vi "ERD_Event_Trigger.vi"(0 ".NET Refnum in":refnum<k24>, 5 "GEA Inputs":T1 {"Destination" format="%.0x"; "Source" format="%.0x"}, 9 "ERD Number":u16, 11 "error in (no error)":errorcluster) -> (4 ".NET Refnum out":refnum<k24>, 15 "error out":errorcluster)   [LabVIEW 2016]
uses:
  Common/LabVIEW GEA2 Toolkit/LabVIEW_GEA2_Toolkit.lvlibp/type defs/Source_Destination.ctl
  Q:/Common/DLLs/GEA3/GeaCommunication.dll
  Common/DLLs/GEA3/GeaCommunication.dll
  Common/LabVIEW GEA2 Toolkit/LabVIEW_GEA2_Toolkit.lvlibp/type defs/ERD Read Data In.ctl
  Common/LabVIEW GEA2 Toolkit/LabVIEW_GEA2_Toolkit.lvlibp/type defs/Data Type.ctl
  Common/LabVIEW GEA2 Toolkit/LabVIEW_GEA2_Toolkit.lvlibp/type defs/ERD Write Data In.ctl
  Common/LabVIEW GEA2 Toolkit/LabVIEW_GEA2_Toolkit.lvlibp
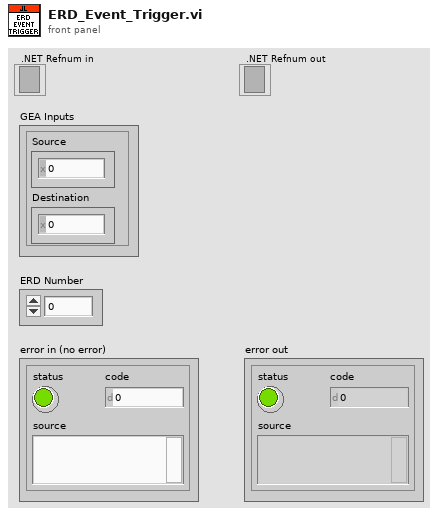
[diagram p1: front panel]
types:
  T1 = typedef "LabVIEW_GEA2_Toolkit.lvlibp/Source_Destination.ctl" = cluster{"Source":u8, "Destination":u8}
  T2 = typedef "LabVIEW_GEA2_Toolkit.lvlibp/ERD Write Data In.ctl" = cluster{"ERD Number":u16, "Data Type":T3, "Data":string}
  T3 = typedef "LabVIEW_GEA2_Toolkit.lvlibp/Data Type.ctl" = enum16{"string", "boolean", "uint8_t", "uint16_t", "uint32_t", "uint64_t", "int8_t", "int16_t", "int32_t", "int64_t"}
  T4 = typedef "LabVIEW_GEA2_Toolkit.lvlibp/ERD Read Data In.ctl" = cluster{"ERD Number":u16, "Data Type":T3}
  T5 = typedef "LabVIEW_GEA2_Toolkit.lvlibp/ERD Read Data Out.ctl" = cluster{"ERD Number":u16, "Data":string}
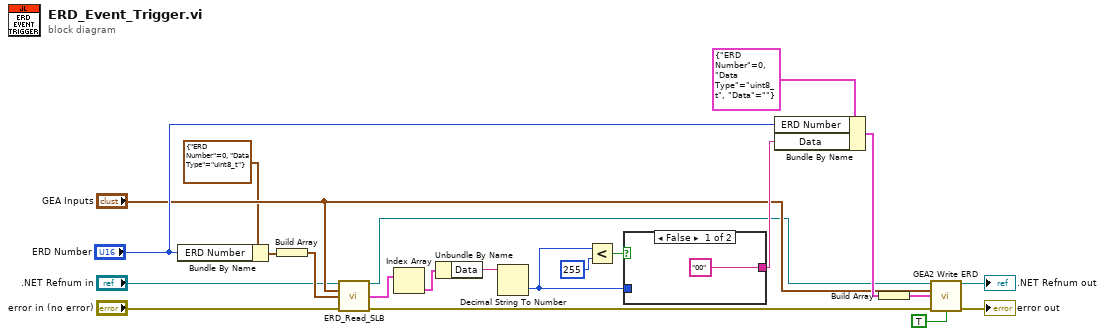
[diagram p0: block diagram]
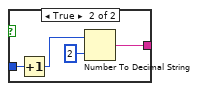
[diagram p2: hidden frame]
diagram:
  n1 = Bundle By Name(cluster=T4 {"ERD Number"=0, "Data Type"=enum."uint8_t"} ("ERD Read Data In"), "ERD Number"="ERD Number") -> (w8:T4)
  n2 = Build Array(w8) -> (w9:T4[])
  n3 = call "ERD_Read_SLB.vi"("GEA2 Reference In"=".NET Refnum in", "GEA Inputs"="GEA Inputs", "Read ERD List"=w9, "Error In"="error in (no error)") -> ("GEA2 Reference Out"=w16:refnum<k24>, "ERD Data Out"=w10:T5[], "Error Out"=w13:errorcluster)  [unwired: 9 in]
  n4 = Index Array(array=w10) -> (element=w11:T5)  [unwired: 1 in]
  n5 = Unbundle By Name(w11) -> ("Data"=w12:string)
  n6 = Decimal String To Number(string=w12) -> (number=w3:i32)  [unwired: 2 in, 1 out]
  n7 = Less?(x=w3, y=255) -> (x < y?=w4:bool)
  n8 = case shown="False" w4 {
    tunnel: ["00" w26] -> w22
    tunnel: w3 -> [_ w25]
    frame False {
    }
    frame True {
      n9 = Increment(x=w25) -> (x+1=w24:i32)
      n10 = Number To Decimal String(number=w24, width (-)=i16 2) -> (decimal integer string=w26:string)
    }
  }
  n11 = Bundle By Name(cluster=T2 {"ERD Number"=0, "Data Type"=enum."uint8_t", "Data"=""} ("ERD Write Data In"), "ERD Number"="ERD Number", "Data"=w22) -> (w19:T2)
  n12 = Build Array(w19) -> (w20:T2[])
  n13 = call "GEA2 Write ERD.vi"("GEA2 Reference In"=w16, "GEA Inputs"="GEA Inputs", "Write ERD List"=w20, "Error In"=w13, "Verify ERD Response?"=TRUE) -> ("GEA2 Reference Out"=→".NET Refnum out":refnum<k24>, "Error Out"=→"error out":errorcluster)  [unwired: 8 in, 1 out]
